vi "Set Sweep Mode.vi"(8 "error in (no error)":errorcluster, 9 "Sweep mode (auto)":T1, 10 "Channel (0: Channel 1)":T2 items=["Channel 1", "Channel 2"], 11 "VISA resource name":refnum<visa-resource-name>) -> (0 "error out":errorcluster, 3 "VISA resource name out":refnum<visa-resource-name>)   [LabVIEW 2009, in "Tektronix AFG 3000 Series.lvlib"]
doc: "Sets the sweep mode of a Tektronix AFG 3000 series function generator to either auto or manual. In auto mode the AFG sweeps continuously; in manual mode, it sweeps once each time it gets a trigger."
uses:
  Tektronix AFG 3000 Series.lvlib
  controls.llb/Channel.ctl
  controls.llb/Sweep Mode.ctl
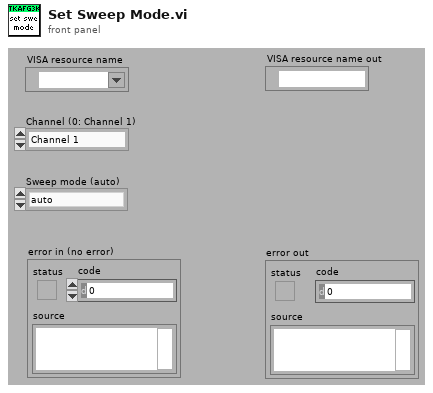
[diagram p1: front panel]
types:
  T1 = typedef "Sweep Mode.ctl" = enum16{"auto", "manual/triggered"}
  T2 = typedef "Channel.ctl" = u16
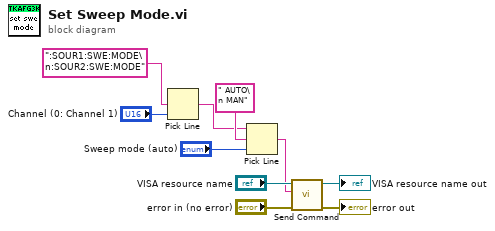
[diagram p0: block diagram]
diagram:
  n1 = Pick Line(multi-line string=":SOUR1:SWE:MODE\n:SOUR2:SWE:MODE", line index="Channel (0: Channel 1)") -> (output string=w4:string)  [unwired: 1 out]
  n2 = Pick Line(string ("")=w4, multi-line string=" AUTO\n MAN", line index="Sweep mode (auto)") -> (output string=w2:string)
  n3 = call "Send Command.vi"("error in (no error)"="error in (no error)", "write buffer"=w2, "VISA resource name"="VISA resource name") -> ("error out"=→"error out":errorcluster, "VISA resource name out"=→"VISA resource name out":refnum<visa-resource-name>)  [unwired: 7 out]
